vi "Read Key (Double).vi"(7 "section":string, 8 "error in (no error)":errorcluster, 9 "default value":dbl format="%.2f", 10 "key":string, 11 "refnum":T1) -> (0 "error out":errorcluster, 1 "value":dbl format="%.2f", 2 "found?":bool, 3 "refnum out":T1)   [LabVIEW 2009]
doc: "Reads a value associated with a key in a specified section from the configuration data identified by <B>refnum</B>. If the key does not exist, the VI returns the default value. You can use this polymorphic VI to read the following types of values from a key: Boolean, double-precision numeric, signed integer, path, string, and unsigned integer. The data type you wire to the <B>default value</B> input determines the polymorphic instance to use."
uses:
  <vilib>/Utility/config.llb/Config Data RefNum.ctl
  <vilib>/Utility/config.llb/NI_LVConfig.lvlib
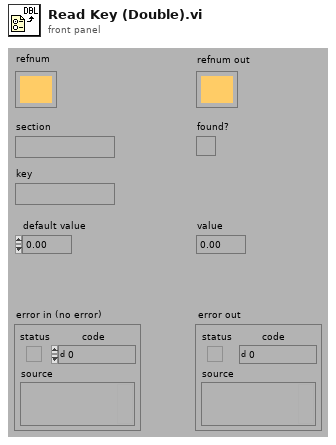
[diagram p1: front panel]
types:
  T1 = typedef "NI_LVConfig.lvlib/Config Data RefNum.ctl" = refnum<k1>
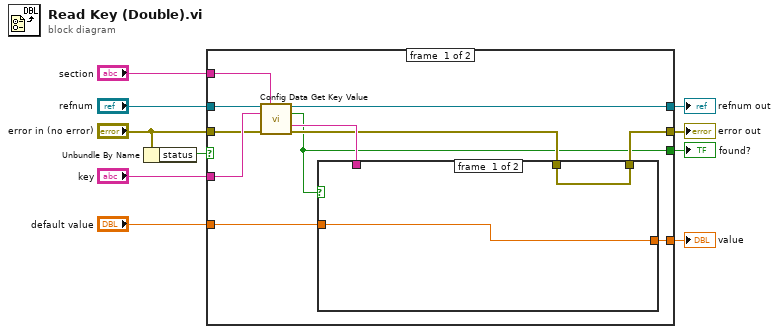
[diagram p0: block diagram]
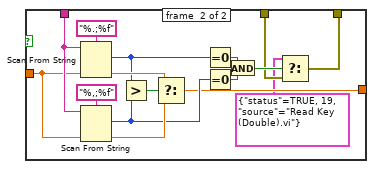
[diagram p2: hidden frame]
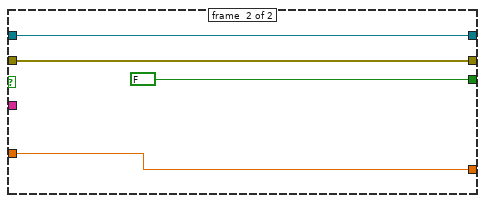
[diagram p3: hidden frame]
diagram:
  n1 = Unbundle By Name("error in (no error)") -> ("status"=w10:bool)
  n2 = case shown="False" w10 {
    tunnel: [w19 w42] -> w9
    tunnel: [w12 w43] -> w8
    tunnel: "refnum" -> [w17 w42]
    tunnel: "error in (no error)" -> [w18 w43]
    tunnel: "section" -> [w21 _]
    tunnel: "key" -> [w20 _]
    tunnel: [w11 FALSE ("section exists?")] -> w7
    tunnel: [w14 w41] -> w6
    tunnel: "default value" -> [w15 w41]
    frame #0 {
      n3 = call "Config Data Get Key Value.vi"("config data"=w17, "section"=w21, "key"=w20, "error in (no error)"=w18) -> ("config data out"=w19:T1, "key exists?"=w11:bool, "key value"=w16:string, "error out"=w13:errorcluster)  [unwired: 6 in, 2 out]
      n4 = case shown="True" w11 {
        tunnel: w16 -> [_ w37]
        tunnel: w15 -> [w22 w36]
        tunnel: [w22 w28] -> w14
        tunnel: w13 -> [w23 w26]
        tunnel: [w23 w24] -> w12
        frame #0 {
        }
        frame #1 {
          n5 = Scan From String(format string="%.;%f" ("Format String"), input string=w37, default 1=w36) -> (offset past scan=w32:u32, output 1=w34:dbl)  [unwired: 2 in, 2 out]
          n6 = Scan From String(format string="%,;%f" ("Format String"), input string=w37, default 1=w36) -> (offset past scan=w30:u32, output 1=w33:dbl)  [unwired: 2 in, 2 out]
          n7 = Greater?(x=w32, y=w30) -> (0:w35:bool)
          n8 = Select(t=w34, s=w35, f=w33) -> (s? t:f=w28:dbl)
          n9 = Equal To 0?(x=w32) -> (x = 0?=w31:bool)
          n10 = Equal To 0?(x=w30) -> (x = 0?=w29:bool)
          n11 = And(x=w31, y=w29) -> (x .and. y?=w27:bool)
          n12 = Select(t=cluster{"status":bool, u16, "source":string} {"status"=TRUE, 19, "source"="Read Key (Double).vi"} ("f"), s=w27, f=w26) -> (s? t:f=w24:errorcluster)
        }
      }
    }
    frame #1 {
    }
  }
  "error out" <- w8
  "refnum out" <- w9
  "value" <- w6
  "found?" <- w7
